vi "Init_Actor_Test.vi"(8 "error in (no error)":errorcluster caption="entrée d'erreur (pas d'erreur)", 11 "Test (Default) en entrée":refnum<class "Actor Test (Default).lvclass">) -> (0 "error out":errorcluster caption="sortie d'erreur", 3 "Test (Default) en sortie":refnum<class "Actor Test (Default).lvclass">)   [LabVIEW 2020, in "Library Core.lvlib" / "Actor Test (Default).lvclass"]
uses:
  Actor Test (Default).lvclass
  Commun VI/TypeDef/Variable Printable.ctl
  Actor Test (Default).lvclass/Actor Test (Default).ctl
  Launch_Actor_Test.vi
  Commun VI/Library Commun.lvlib
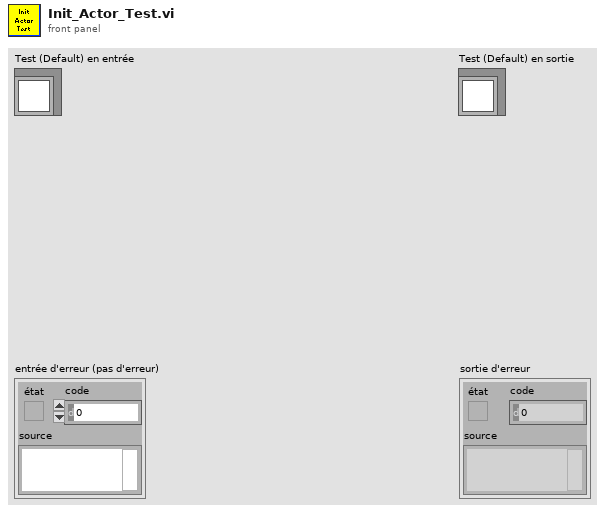
[diagram p1: front panel]
types:
  T1 = typedef "Variable Printable.ctl" = string
  T2 = enum16{"Get Variable", "Get All Variables", "Set Variable", "Delete Variable", "Delete All Variable"}
  T3 = enum16{"Get Loop Sequence", "Reset", "Set Loop Sequence"}
  T4 = enum16{"Get Actor Class", "Set Actor object", "Get Actor object", "List Actor", "Init"}
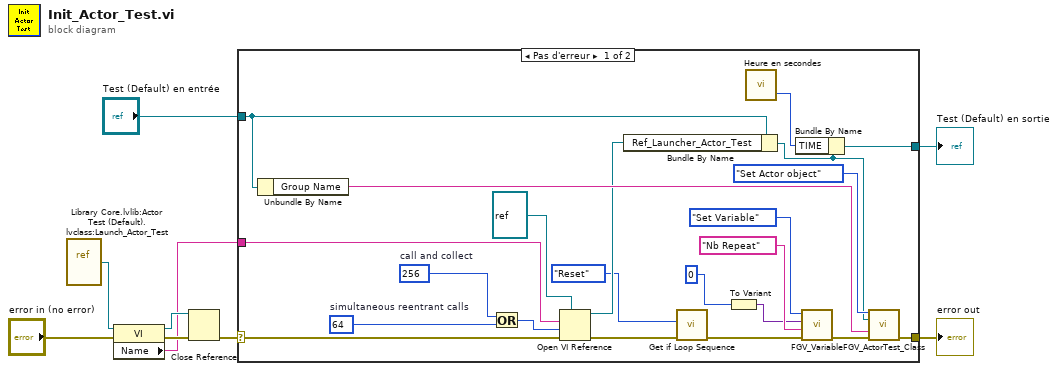
[diagram p0: block diagram]
diagram:
  n1 = vi-ref "Library Core.lvlib:Actor Test (Default).lvclass:Launch_Actor_Test.vi"() -> (w1:refnum<vi>)
  n2 = property class="VI"(reference=w1, error in="error in (no error)") -> (reference out=w9:refnum<vi>, error out=w8:errorcluster, "Name"=w7:string)
  n3 = Close Reference(reference=w9, error in (no error)=w8) -> (error out=w6:errorcluster)
  n4 = case shown="Pas d'erreur" w6 {
    selector: w6 -> [w18 w33]
    tunnel: [w30 w33] -> w2
    tunnel: [w25 w32] -> w4
    tunnel: "Test (Default) en entrée" -> [w28 w32]
    tunnel: w7 -> [w31 _]
    frame No Error {
      w22 = 64  # simultaneous reentrant calls
      w21 = 256  # call and collect
      n5 = Unbundle By Name(w28) -> ("Group Name"=w27:string)
      n6 = Or(x=w21, y=w22) -> (x .or. y?=w20:i32)
      n7 = Open VI Reference(type specifier VI Refnum (for type only)=refnum<vi> refnum ("spécificateur de type du refnum de VI (pour type seulement)"), vi path=w31, options=w20, error in (no error)=w18) -> (vi reference=w19:refnum<vi>, error out=w17:errorcluster)  [unwired: 2 in]
      n8 = Bundle By Name(cluster=w28, "Ref_Launcher_Actor_Test"=w19) -> (w26:refnum<class "Actor Test (Default).lvclass">)
      n9 = call "Get if Loop Sequence.vi"("error in (no error)"=w17, "Function"=T3."Reset") -> ("error out"=w13:errorcluster)  [unwired: 8 in, 1 out]
      n10 = To Variant(anything=0) -> (Variant=w10:variant)
      n11 = call "Heure en secondes.vi"() -> ("Heure en milisecondes"=w24:u32)  [unwired: 2 in, 1 out]
      n12 = Bundle By Name(cluster=w26, "TIME"=w24) -> (w25:refnum<class "Actor Test (Default).lvclass">)
      n13 = call "FGV_Variable.vi"("error in (no error)"=w13, "Variable"=T1 "Nb Repeat", "Data In"=w10, "Function"=T2."Set Variable") -> ("error out"=w12:errorcluster)  [unwired: 5 in, 2 out]
      n14 = call "FGV_ActorTest_Class.vi"("Action"=T4."Set Actor object", "Actor Test"=w26, "Group Name"=w27, "error in (no error)"=w12) -> ("error out"=w30:errorcluster)  [unwired: 8 in, 3 out]
    }
    frame Error {
    }
  }
  "error out" <- w2
  "Test (Default) en sortie" <- w4
